vi "Qrcode YGB.vi"() -> ()   [LabVIEW 2019]
uses:
  <vilib>/userDefined/High Color/IMAQdx.ctl
  <vilib>/vision/driver/NI_Vision_Acquisition_Software.lvlib
  <vilib>/vision/NI_Vision_Development_Module.lvlib
panel:
  out "Blue":bool
  out "Green":bool
  out "Yellow":bool
  out "code 3":string
  out "code 2":string
  out "code 1":string
  in  "Session In":T1
  out "Found?":bool
  out "Image":T2(plugin-control)
  out "Code":string
  out "Code Array":string[](array[string])
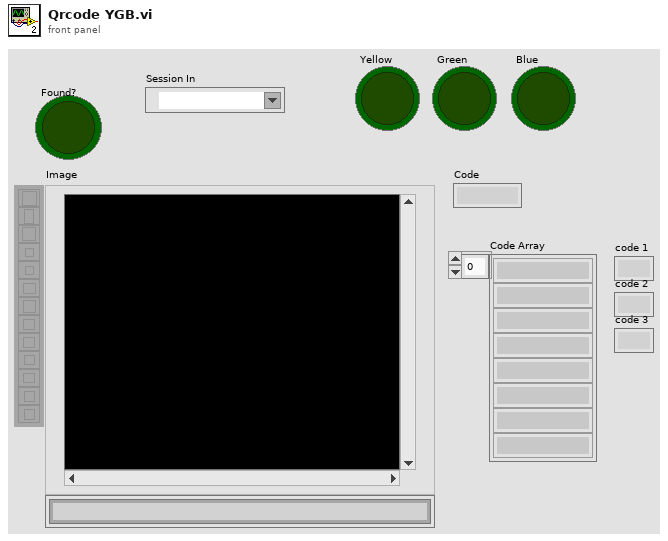
[diagram p1: front panel]
types:
  T1 = typedef "IMAQdx.ctl" = refnum<k21>
  T2 = typedef "IMAQ Image.ctl" = refnum<image>
  T3 = typedef "Image Type" = u32
  T4 = typedef "QR Code Report.ctl" = cluster{"Found?":bool, "Data":string, "Bounding Box":cluster{"x":sgl, "y":sgl}[], "Errors Corrected":u32, "Dimensions (Rows/Cols)":u32, "Version":u32, "QR Model":T5, "Stream Mode":T6, "Barcode Polarity":T7, "Mirrored?":bool, "Append Stream Position":u32, "Size of Append Stream":u32, "First EAN-128 ID":i32, "First Alternate Language ID":i32, "Append Stream ID":u32, "Minimum Edge Strength":u32, "Demodulation Mode":T8, "Cell Sample Size":T9, "Cell Filter Mode":T10}
  T5 = typedef "QR Code Model Type.ctl" = i32
  T6 = typedef "QR Code Stream Mode Type.ctl" = i32
  T7 = typedef "Data Matrix Polarity.ctl" = i32
  T8 = typedef "Demodulation Mode.ctl" = i32
  T9 = typedef "Cell Sample Size.ctl" = i32
  T10 = typedef "Cell Filter Mode.ctl" = i32
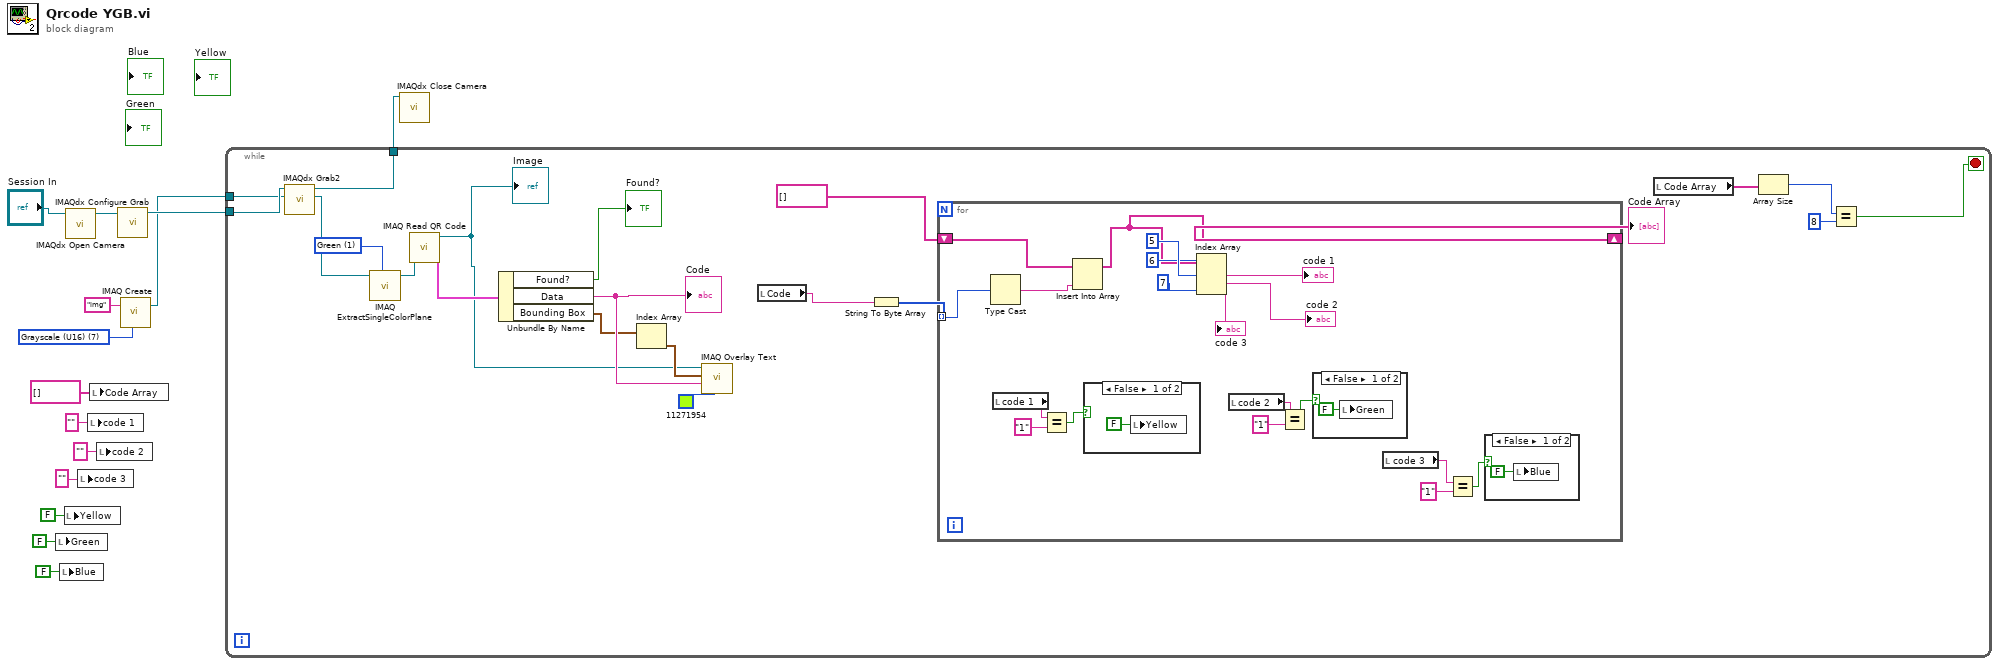
[diagram p0: block diagram]
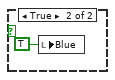
[diagram p2: hidden frame]
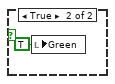
[diagram p3: hidden frame]
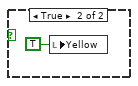
[diagram p4: hidden frame]
diagram:
  w9 = T3 7 items=["Grayscale (U8)", "Grayscale (I16)", "Grayscale (SGL)", "Complex (CSG)", "RGB (U32)", "HSL (U32)", "RGB (U64)", "Grayscale (U16)"] ("Image Type")
  n1 = local write "Green"(FALSE ("Green")) -> ()
  n2 = local write "Blue"(FALSE ("Blue")) -> ()
  n3 = local write "Yellow"(FALSE ("Yellow")) -> ()
  n4 = call <vilib>:"IMAQdx Open Camera.vi"("Session In"="Session In") -> ("Session Out"=w13:T1)  [unwired: 9 in, 1 out]
  n5 = local write "code 3"("" ("code 3")) -> ()
  n6 = local write "code 1"("" ("code 1")) -> ()
  n7 = local write "Code Array"(string[] [] ("Code Array")) -> ()
  n8 = local write "code 2"("" ("code 2")) -> ()
  n9 = call <vilib>:"IMAQdx Configure Grab.vi"("Session In"=w13) -> ("Session Out"=w11:T1)  [unwired: 9 in, 1 out]
  n10 = call "IMAQ Create"("Image Name"="img", "Image Type"=w9) -> ("New Image"=w8:T2)  [unwired: 3 in, 1 out]
  n11 = while {
    tunnel: [w35] -> w12
    tunnel: w11 -> [w34]
    tunnel: w8 -> [w33]
    stop <- w18 stop-if-true
    w30 = 1 items=["Red", "Green", "Blue", "Hue", "Saturation", "Luminance", "Value", "Intensity"] ("Color Plane")
    n12 = call <vilib>:"IMAQdx Grab2.vi"("Image In"=w33, "Session In"=w34) -> ("Image Out"=w32:T2, "Session Out"=w35:T1)  [unwired: 6 in, 2 out]
    n13 = call "IMAQ ExtractSingleColorPlane"("Color Plane"=w30, "Image Src"=w32) -> ("Image Dst Out"=w31:T2)  [unwired: 8 in, 1 out]
    n14 = call "IMAQ Read QR Code"("Image"=w31) -> ("QR Code Report"=w29:T4, "Image (duplicate)"=w23:T2)  [unwired: 7 in, 2 out]
    "Image" <- w23
    n15 = Unbundle By Name(w29) -> ("Found?"=→"Found?":bool, "Data"=w26:string, "Bounding Box"=w24:cluster{"x":sgl, "y":sgl}[])
    "Code" <- w26
    n16 = Index Array(array=w24) -> (element=w27:cluster{"x":sgl, "y":sgl})  [unwired: 1 in]
    n17 = call "IMAQ Overlay Text"("Text Color (black)"=u32 11271954, "String"=w26, "Origin"=w27, "Image"=w23) -> ()  [unwired: 6 in, 2 out]
    n18 = local read "Code"() -> (w19:string)
    n19 = String To Byte Array(string=w19) -> (unsigned byte array=w22:u8[])
    n20 = for {
      tunnel: w22 -> [w54] mode=indexing
      shift-right: [w48] -> w20
      shift-left: string[] [] -> [w53]
      n21 = Type Cast(x=w54) -> (*(type *) &x=w52:string)  [unwired: 1 in]
      n22 = local read "code 1"() -> (w43:string)
      n23 = Equal?(x=w43, y="1") -> (x = y?=w44:bool)
      n24 = Insert Into Array(array=w53, new element=w52) -> (w48:string[])  [unwired: 1 in]
      n25 = case shown="False" w44 {
        frame False {
          n26 = local write "Yellow"(FALSE ("Yellow")) -> ()
        }
        frame True {
          n27 = local write "Yellow"(TRUE ("Yellow")) -> ()
        }
      }
      n28 = Index Array(array=w48, index #1=5 ("index"), index #2=6 ("index"), index #3=7 ("index")) -> (element #1=→"code 1":string, element #2=→"code 2":string, element #3=→"code 3":string)
      n29 = local read "code 2"() -> (w41:string)
      n30 = Equal?(x=w41, y="1") -> (x = y?=w37:bool)
      n31 = case shown="False" w37 {
        frame False {
          n32 = local write "Green"(FALSE ("Green")) -> ()
        }
        frame True {
          n33 = local write "Green"(TRUE ("Green")) -> ()
        }
      }
      n34 = local read "code 3"() -> (w40:string)
      n35 = Equal?(x=w40, y="1") -> (x = y?=w36:bool)
      n36 = case shown="False" w36 {
        frame False {
          n37 = local write "Blue"(FALSE ("Blue")) -> ()
        }
        frame True {
          n38 = local write "Blue"(TRUE ("Green")) -> ()
        }
      }
    }
    "Code Array" <- w20
    n39 = local read "Code Array"() -> (w17:string[])
    n40 = Array Size(array=w17) -> (size(s)=w16:i32)
    n41 = Equal?(x=w16, y=8) -> (x = y?=w18:bool)
  }
  n42 = call <vilib>:"IMAQdx Close Camera.vi"("Session In"=w12) -> ()  [unwired: 10 in, 1 out]
